vi "StartHarvest.vi"(8 "error in (no error)":errorcluster, 11 "Controller in":refnum<class "Controller.lvclass">) -> (0 "error out":errorcluster, 3 "Controller out":refnum<class "Controller.lvclass">)   [LabVIEW 2022 SP3, in "Controller.lvlib" / "Controller.lvclass"]
uses:
  Controller.lvclass
  Controller.lvclass/Controller.ctl
  <vilib>/ActorFramework/Message Enqueuer/Message Enqueuer.lvclass/Message Enqueuer.ctl
  <vilib>/ActorFramework/Message Enqueuer/Enqueue.vi
  UserInterface/UserInterface Messages/Reset UI Msg/Reset UI Msg.lvclass
  C:/Program Files/National Instruments/LabVIEW 2022/vi.lib/ActorFramework/Message/Message.lvclass
  PLCHandler/PLCHandler Messages/Wakeup Msg/Wakeup Msg.lvclass
  <vilib>/ActorFramework/Message Priority Queue/Priority Enqueue.vi
  <vilib>/ActorFramework/Message Enqueuer/Message Enqueuer.lvclass
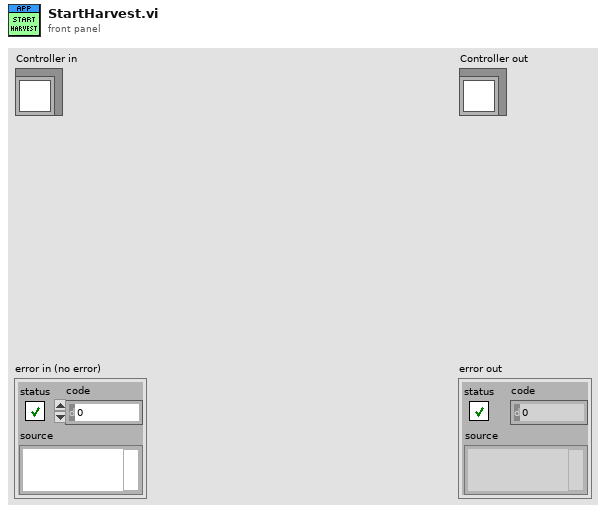
[diagram p1: front panel]
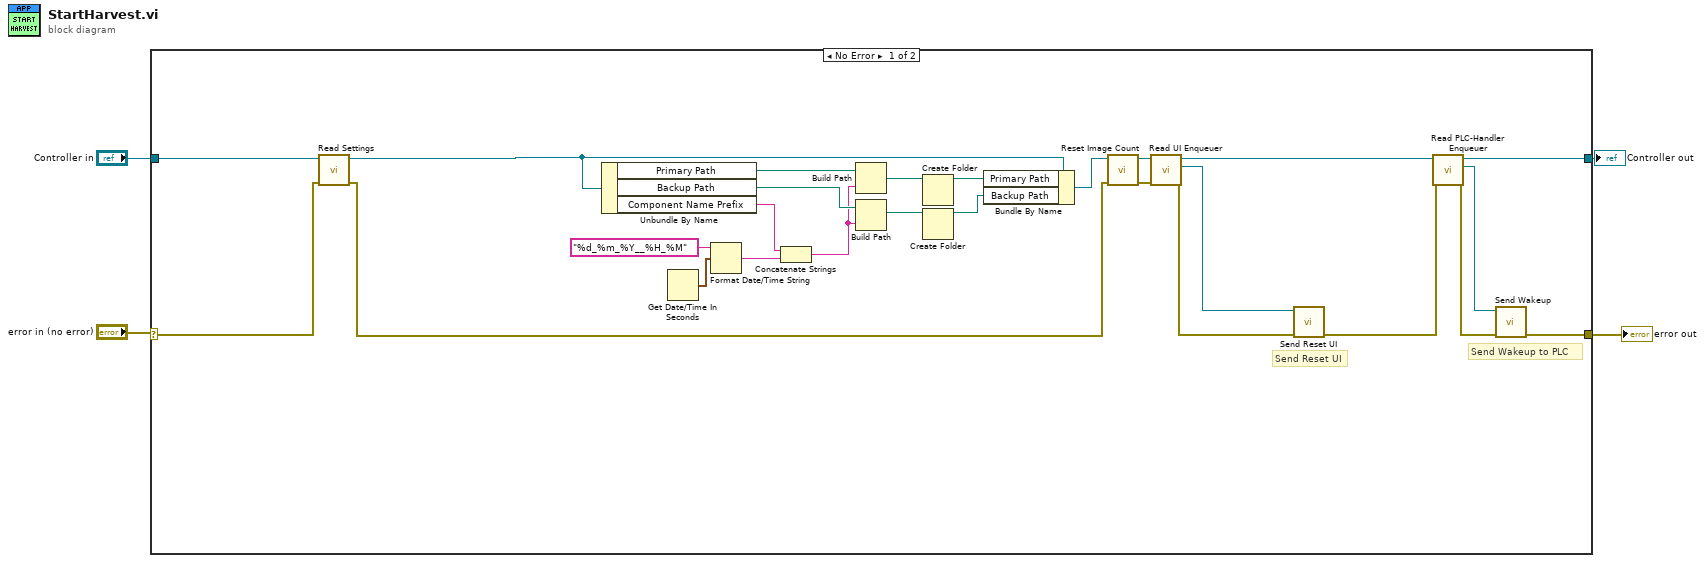
[diagram p0: block diagram]
diagram:
  n1 = case shown="No Error" "error in (no error)" {
    selector: "error in (no error)" -> [w6 w31]
    tunnel: [w30 w31] -> w4
    tunnel: [w29 w32] -> w3
    tunnel: "Controller in" -> [w8 w32]
    frame No Error {
      # "Send Wakeup to PLC"
      # "Send Reset UI"
      n2 = call "Read Settings.vi"("error in"=w6, "Controller in"=w8) -> ("error out"=w5:errorcluster, "Controller out"=w7:refnum<class "Controller.lvclass">)  [unwired: 7 in, 1 out]
      n3 = Unbundle By Name(w7) -> ("Primary Path"=w22:path, "Backup Path"=w21:path, "Component Name Prefix"=w11:string)
      n4 = Get Date/Time In Seconds() -> (seconds since 1Jan1904=w18:timestamp)
      n5 = Format Date/Time String(time format string (%c)="%d_%m_%Y__%H_%M", seconds (now)=w18) -> (date/time string=w17:string)  [unwired: 1 in]
      n6 = Concatenate Strings(w11, w17) -> (w20:string)
      n7 = Build Path(base path=w22, name or relative path=w20) -> (appended path=w15:path)
      n8 = Build Path(base path=w21, name or relative path=w20) -> (appended path=w13:path)
      n9 = Create Folder(path (use dialog)=w15) -> (created path=w14:path)  [unwired: 2 in, 2 out]
      n10 = Create Folder(path (use dialog)=w13) -> (created path=w12:path)  [unwired: 2 in, 2 out]
      n11 = Bundle By Name(cluster=w7, "Primary Path"=w14, "Backup Path"=w12) -> (w16:refnum<class "Controller.lvclass">)
      n12 = call "Reset Image Count.vi"("error in (no error)"=w5, "Controller in"=w16) -> ("error out"=w28:errorcluster, "Controller out"=w27:refnum<class "Controller.lvclass">)  [unwired: 8 in]
      n13 = call "Read UI Enqueuer.vi"("error in (no error)"=w28, "Controller in"=w27) -> ("error out"=w9:errorcluster, "Actor Framework:Message Enqueuer"=w10:refnum<class "Message Enqueuer.lvclass">, "Controller out"=w25:refnum<class "Controller.lvclass">)  [unwired: 7 in]
      n14 = call "Send Reset UI.vi"("error in (no error)"=w9, "Message Enqueuer"=w10) -> ("error out"=w23:errorcluster)  [unwired: 8 in, 1 out]
      n15 = call "Read PLC-Handler Enqueuer.vi"("error in (no error)"=w23, "Controller in"=w25) -> ("error out"=w24:errorcluster, "Actor Framework:Message Enqueuer"=w26:refnum<class "Message Enqueuer.lvclass">, "Controller out"=w29:refnum<class "Controller.lvclass">)  [unwired: 7 in]
      n16 = call "Send Wakeup.vi"("error in (no error)"=w24, "Message Enqueuer"=w26) -> ("error out"=w30:errorcluster)  [unwired: 8 in, 1 out]
    }
    frame Error {
    }
  }
  "error out" <- w4
  "Controller out" <- w3
